vi "TimerStop.vi"(11 "Start Zeit":dbl) -> (3 "String":string)   [LabVIEW 2013, in "EMV-Test.lvlib"]
uses:
  lib/EMV-Test.lvlib
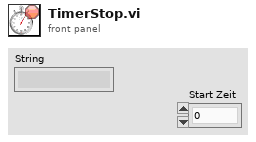
[diagram p1: front panel]
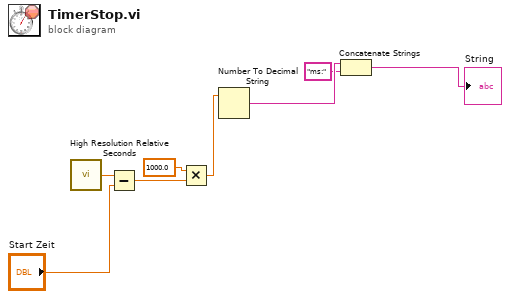
[diagram p0: block diagram]
diagram:
  n1 = call <vilib>:"High Resolution Relative Seconds.vi"() -> ("relative seconds"=w5:dbl)
  n2 = Subtract(x=w5, y="Start Zeit") -> (x-y=w6:dbl)
  n3 = Multiply(x=1000.0, y=w6) -> (x*y=w8:dbl)
  n4 = Number To Decimal String(number=w8) -> (decimal integer string=w3:string)  [unwired: 1 in]
  n5 = Concatenate Strings(w3, "ms:" ("string")) -> (→"String":string)
